vi "niFpgaPID_PDStatelessCore.vi"(0 "errors":T3, 1 "reset? (F)":bool, 5 "enable bumpless transfer? (F)":bool, 7 "manual control":T6, 11 "state in":T2, 12 "gains":T4 {"filter coefficient" min=0 max=1; "proportional gain" step=0.125}, 13 "output range":T5={"output high (Inf)"=inf, "output low (-Inf)"=-inf}) -> (4 "output":sgl, 8 "actions":T1, 15 "state out":T2)   [LabVIEW 2017]
uses:
  <vilib>/rvi/Analysis/control/PID/Typedef/niFpgaPID_ManualControl.ctl
  <vilib>/rvi/Analysis/control/PID/Typedef/niFpgaPID_OutputRange.ctl
  <vilib>/rvi/Analysis/control/PID/Typedef/niFpgaPID_PDGains.ctl
  <vilib>/rvi/Analysis/control/PID/Typedef/niFpgaPID_PDErrors.ctl
  <vilib>/rvi/Analysis/control/PID/Typedef/niFpgaPID_PDState.ctl
  <vilib>/rvi/Analysis/control/PID/Typedef/niFpgaPID_PDActions.ctl
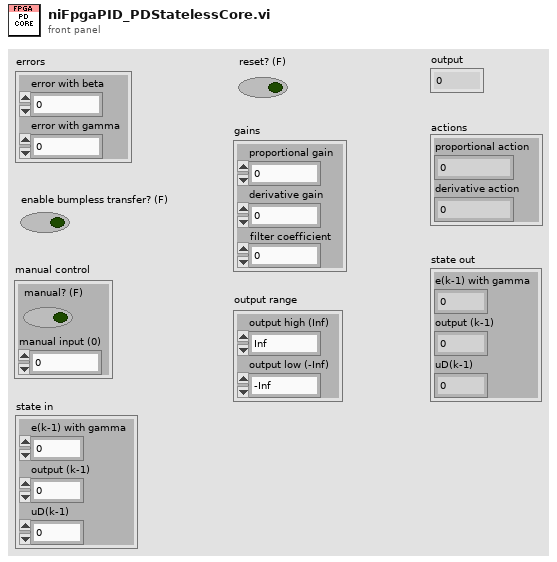
[diagram p1: front panel]
types:
  T1 = typedef "niFpgaPID_PDActions.ctl" = cluster{"proportional action":sgl, "derivative action":sgl}
  T2 = typedef "niFpgaPID_PDState.ctl" = cluster{"e(k-1) with gamma":sgl, "output (k-1)":sgl, "uD(k-1)":sgl}
  T3 = typedef "niFpgaPID_PDErrors.ctl" = cluster{"error with beta":sgl, "error with gamma":sgl}
  T4 = typedef "niFpgaPID_PDGains.ctl" = cluster{"proportional gain":sgl, "derivative gain":sgl, "filter coefficient":sgl}
  T5 = typedef "niFpgaPID_OutputRange.ctl" = cluster{"output high (Inf)":sgl, "output low (-Inf)":sgl}
  T6 = typedef "niFpgaPID_ManualControl.ctl" = cluster{"manual? (F)":bool, "manual input (0)":sgl}
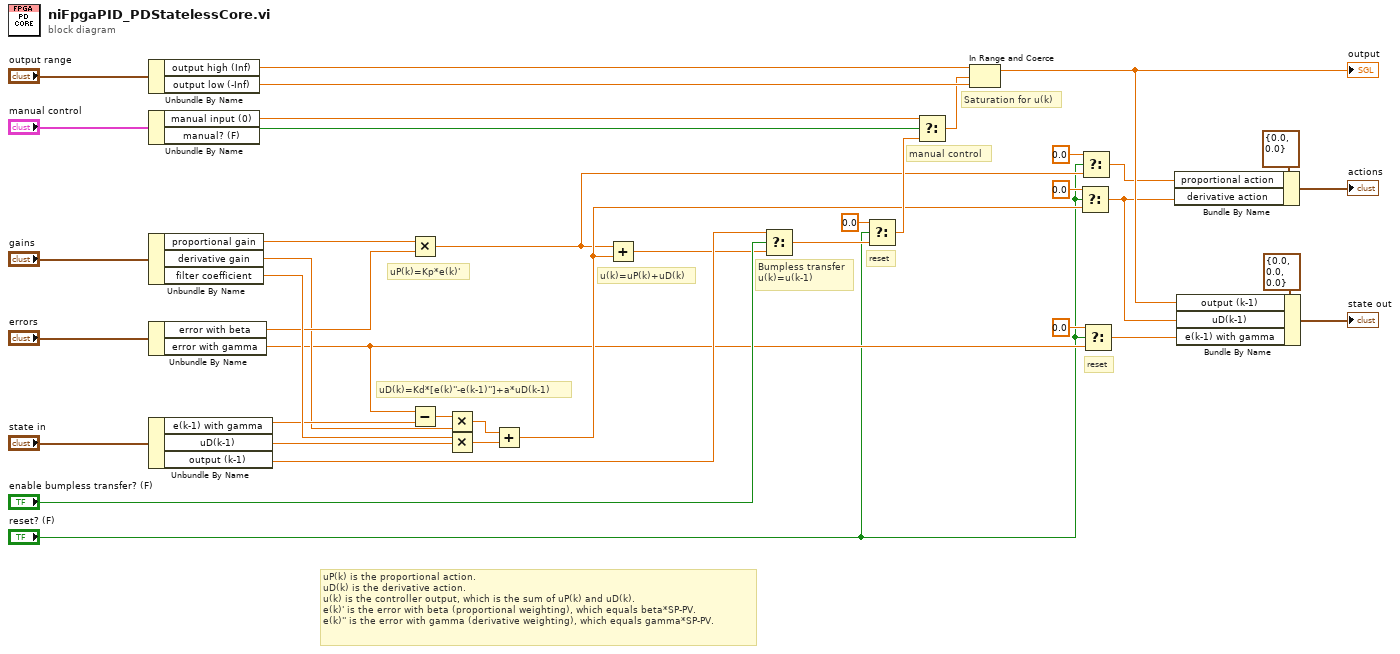
[diagram p0: block diagram]
diagram:
  # "uP(k) is the proportional action.\nuD(k) is the derivative action.\nu(k) is the controller output, which is the sum of uP(k) and uD(k).\ne(k)' is the error with beta (proportional weighting), which equals beta*SP-PV.\ne(k)'' is the error with gamma (derivative weighting), which equals gamma*SP-PV."
  # "manual control"
  # "reset"
  # "reset"
  # "Bumpless transfer\nu(k)=u(k-1)"
  # "Saturation for u(k)"
  # "u(k)=uP(k)+uD(k)"
  # "uD(k)=Kd*[e(k)''-e(k-1)'']+a*uD(k-1)"
  # "uP(k)=Kp*e(k)'"
  n1 = Unbundle By Name("output range") -> ("output high (Inf)"=w40:sgl, "output low (-Inf)"=w39:sgl)
  n2 = Unbundle By Name("manual control") -> ("manual input (0)"=w30:sgl, "manual? (F)"=w29:bool)
  n3 = Unbundle By Name("gains") -> ("proportional gain"=w19:sgl, "derivative gain"=w16:sgl, "filter coefficient"=w38:sgl)
  n4 = Unbundle By Name("errors") -> ("error with beta"=w18:sgl, "error with gamma"=w3:sgl)
  n5 = Unbundle By Name("state in") -> ("e(k-1) with gamma"=w31:sgl, "uD(k-1)"=w37:sgl, "output (k-1)"=w17:sgl)
  n6 = Multiply(x=w19, y=w18) -> (x*y=w7:sgl)
  n7 = Subtract(x=w3, y=w31) -> (x-y=w36:sgl)
  n8 = Multiply(x=w36, y=w16) -> (x*y=w35:sgl)
  n9 = Multiply(x=w38, y=w37) -> (x*y=w34:sgl)
  n10 = Add(x=w35, y=w34) -> (x+y=w9:sgl)
  n11 = Add(x=w7, y=w9) -> (x+y=w13:sgl)
  n12 = Select(t=w17, s="enable bumpless transfer? (F)", f=w13) -> (s? t:f=w20:sgl)
  n13 = Select(t=sgl 0.0 ("f"), s="reset? (F)", f=w20) -> (s? t:f=w27:sgl)
  n14 = Select(t=w30, s=w29, f=w27) -> (s? t:f=w12:sgl)
  n15 = In Range and Coerce(upper limit=w40, x=w12, lower limit=w39) -> (coerced(x)=w11:sgl)  [unwired: 1 out]
  "output" <- w11
  n16 = Select(t=sgl 0.0 ("f"), s="reset? (F)", f=w9) -> (s? t:f=w5:sgl)
  n17 = Select(t=sgl 0.0 ("f"), s="reset? (F)", f=w7) -> (s? t:f=w6:sgl)
  n18 = Select(t=sgl 0.0 ("f"), s="reset? (F)", f=w3) -> (s? t:f=w2:sgl)
  n19 = Bundle By Name(cluster=T1 {"proportional action"=0.0, "derivative action"=0.0} ("actions"), "proportional action"=w6, "derivative action"=w5) -> (→"actions":T1)
  n20 = Bundle By Name(cluster=T2 {"e(k-1) with gamma"=0.0, "output (k-1)"=0.0, "uD(k-1)"=0.0} ("state"), "output (k-1)"=w11, "uD(k-1)"=w5, "e(k-1) with gamma"=w2) -> (→"state out":T2)
